vi "Start_SR830.vi"(0 "Lock-in Reference":u16, 1 "VI-Pfad":path=path "E:/CryoTUM-Software/16T-Magnet_Ultimate-Control_Version_2-0/LS370Monitor.vi") -> ()   [LabVIEW 2018]
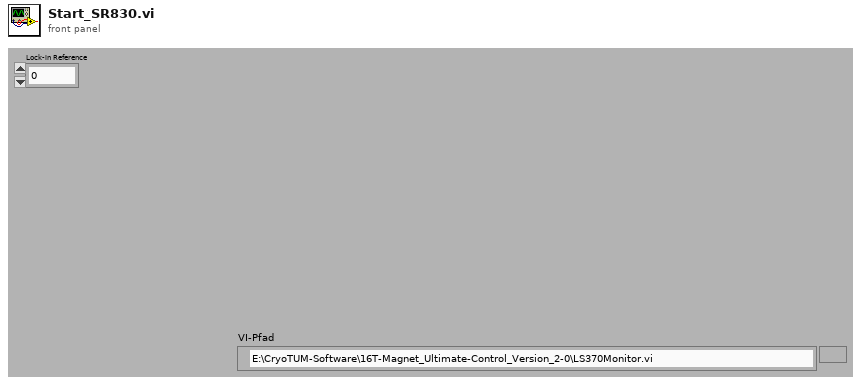
[diagram p1: front panel]
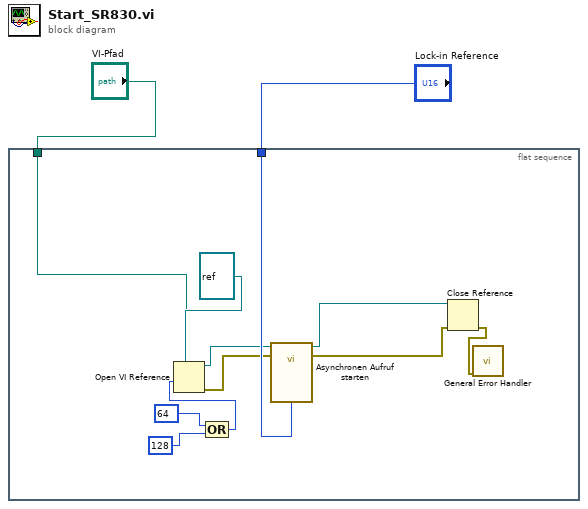
[diagram p0: block diagram]
diagram:
  n1 = flat-sequence {
    tunnel: "VI-Pfad" -> [w3]
    tunnel: "Lock-in Reference" -> [w13]
    frame #0 {
      n2 = Compound Arithmetic op=OR(64 ("options"), 128 ("options")) -> (w5:i32)
      n3 = Open VI Reference ("VI-Referenz öffnen")(type specifier VI Refnum (for type only)=refnum<vi> refnum ("vi reference"), vi path=w3, options=w5) -> (vi reference=w12:refnum<vi>, error out=w11:errorcluster)  [unwired: 3 in]
      n4 = call-by-ref "Asynchronen Aufruf starten"(reference=w12, error in=w11, "Lock-in Reference"=w13) -> (reference out=w10:refnum<vi>, error out=w9:errorcluster)
      n5 = Close Reference(reference=w10, error in (no error)=w9) -> (error out=w8:errorcluster)
      n6 = call <vilib>:"General Error Handler.vi"("error in (no error)"=w8) -> ()  [unwired: 10 in, 5 out]
    }
  }
